vi "ReadJSONImageAcquisitionParameters.vi"(8 "error in":errorcluster, 10 "Camera ID":string="0", 11 "file path (use dialog)":path) -> (0 "error out":errorcluster, 3 "Camera parameters":T1 {"Camera parameters"."Image Type" items=["Grayscale (U8)", "Grayscale (I16)", "Grayscale (SGL)", "Complex (CSG)", "RGB (U32)", "HSL (U32)", "RGB (U64)", "Grayscale (U16)"]})   [LabVIEW 2019, in "Image Acquisition.lvlib" / "Image Acquisition.lvclass"]
uses:
  Image Acquisition.lvclass
  <vilib>/userdefined/High Color/IMAQdx.ctl
  <vilib>/vision/driver/IMAQdx.llb/IMAQdx Acquisition Mode.ctl
  <vilib>/vision/driver/IMAQdx.llb/IMAQdx Buffer Number Mode.ctl
  TypeDefs/Image Acquisition Parameters JSON.ctl
  TypeDefs/Image Acquisition Parameters.ctl
panel:
  out "VCluster\n out":variant
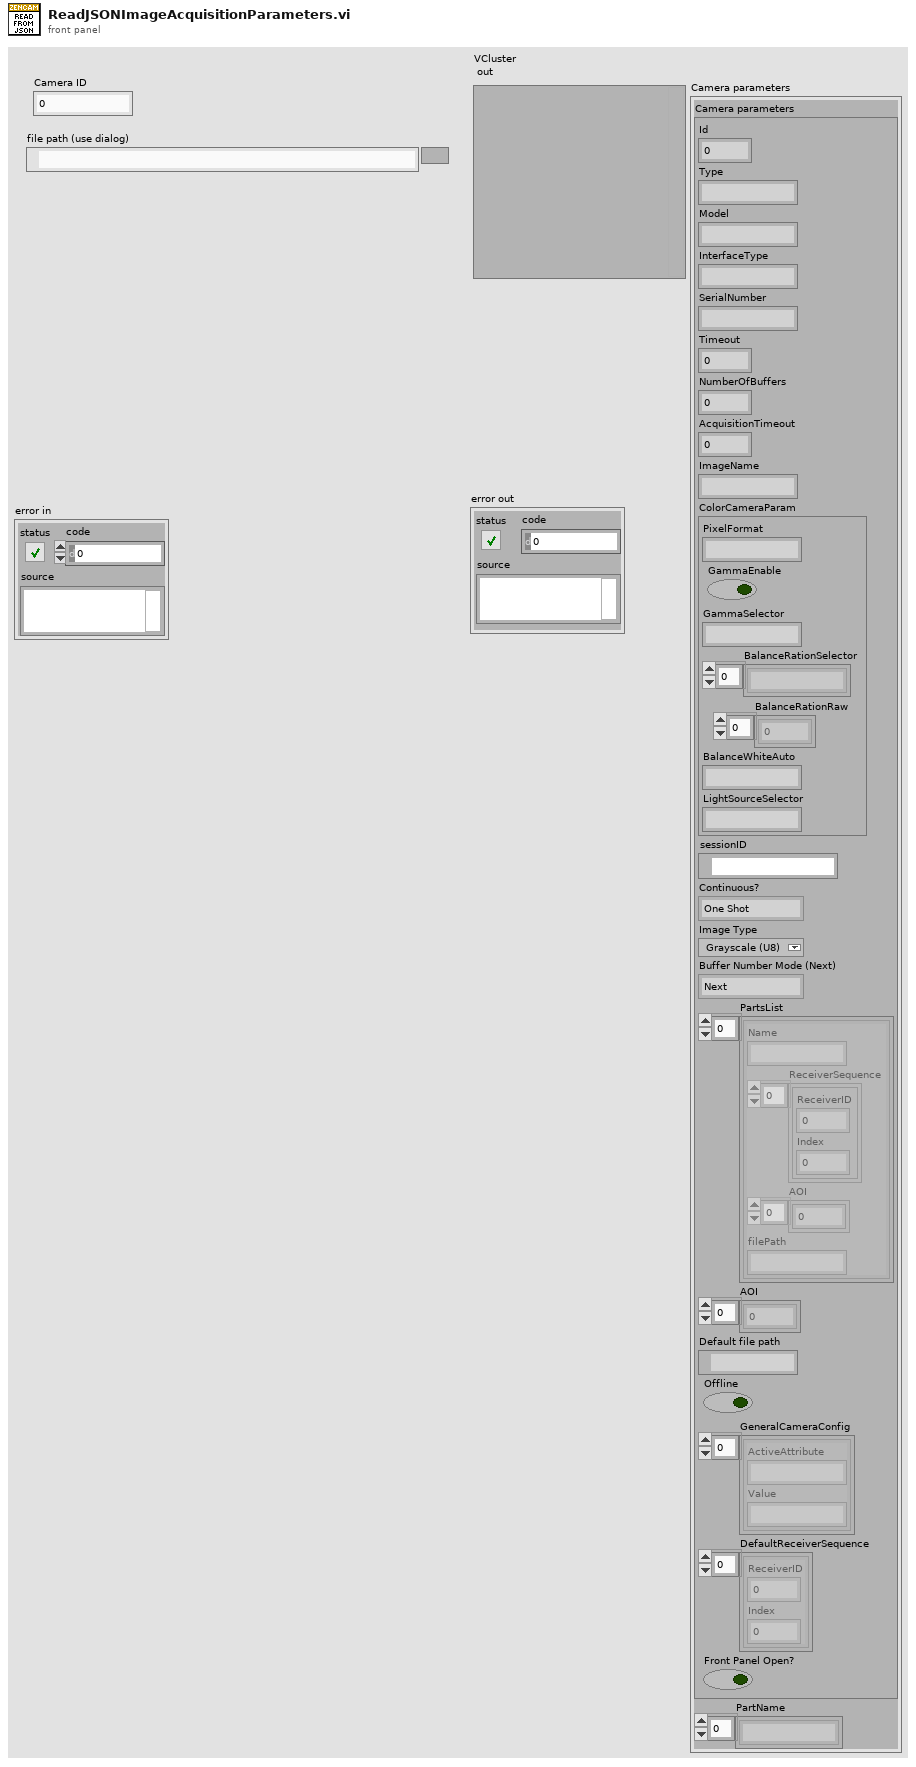
[diagram p1: front panel]
types:
  T1 = typedef "Image Acquisition.lvlib/Image Acquisition.lvclass/Image Acquisition Parameters.ctl" = cluster{"Camera parameters":cluster{"Id":i32, "Type":string, "Model":string, "InterfaceType":string, "SerialNumber":string, "Timeout":i32, "NumberOfBuffers":i32, "AcquisitionTimeout":i32, "ImageName":string, "ColorCameraParam":cluster{"PixelFormat":string, "GammaEnable":bool, "GammaSelector":string, "BalanceRationSelector":string[], "BalanceRationRaw":i32[], "BalanceWhiteAuto":string, "LightSourceSelector":string}, "sessionID":T2, "Continuous?":T3, "Image Type":T4, "Buffer Number Mode (Next)":T5, "PartsList":cluster{"Name":string, "ReceiverSequence":cluster{"ReceiverID":dbl, "Index":dbl}[], "AOI":i32[], "filePath":string}[], "AOI ":i32[], "Default file path":path, "Offline":bool, "GeneralCameraConfig":cluster{"ActiveAttribute":string, "Value":string}[], "DefaultReceiverSequence":cluster{"ReceiverID":dbl, "Index":dbl}[], "Front Panel Open?":bool}, "PartName":string[]}
  T2 = typedef "IMAQdx.ctl" = refnum<k21>
  T3 = typedef "NI_Vision_Acquisition_Software.lvlib/IMAQdx Acquisition Mode.ctl" = enum32{"One Shot", "Continuous"}
  T4 = typedef "Image Type" = u32
  T5 = typedef "NI_Vision_Acquisition_Software.lvlib/IMAQdx Buffer Number Mode.ctl" = enum32{"Next", "Last", "Buffer Number", "Every", "Last New"}
  T6 = typedef "Image Acquisition.lvlib/Image Acquisition.lvclass/Image Acquisition Parameters JSON.ctl" = cluster{"Image Acquisition Paramters":cluster{"Id":i32, "SessionID":string, "Type":string, "Model":string, "InterfaceType":string, "SerialNumber":string, "Timeout":i32, "GeneralCameraConfig":cluster{"ActiveAttribute":string, "Value":string}[], "DefaultAOI":i32[], "DefaultReceiverSequence":cluster{"ReceiverID":i32, "Index":i32}[], "DefaultfileName":string, "Continuous":i32, "NumberOfBuffers":i32, "BufferNumberMode":i32, "acquisitionTimeout":i32, "ImageType":i32, "Offline":bool, "FrontPanelOpen":bool, "ColorCameraParam":cluster{"PixelFormat":string, "GammaEnable":bool, "GammaSelector":string, "BalanceRationSelector":string[], "BalanceRationRaw":i32[], "BalanceWhiteAuto":string, "LightSourceSelector":string}, "PartsList":cluster{"Name":string, "ReceiverSequence":cluster{"ReceiverID":i32, "Index":i32}[], "AOI":i32[], "filePath":string}[]}, "PartName":string[]}
  T7 = cluster{"ActiveAttribute":string, "Value":string}[]
  T8 = cluster{"PixelFormat":string, "GammaEnable":bool, "GammaSelector":string, "BalanceRationSelector":string[], "BalanceRationRaw":i32[], "BalanceWhiteAuto":string, "LightSourceSelector":string}
  T9 = cluster{"Name":string, "ReceiverSequence":cluster{"ReceiverID":i32, "Index":i32}[], "AOI":i32[], "filePath":string}[]
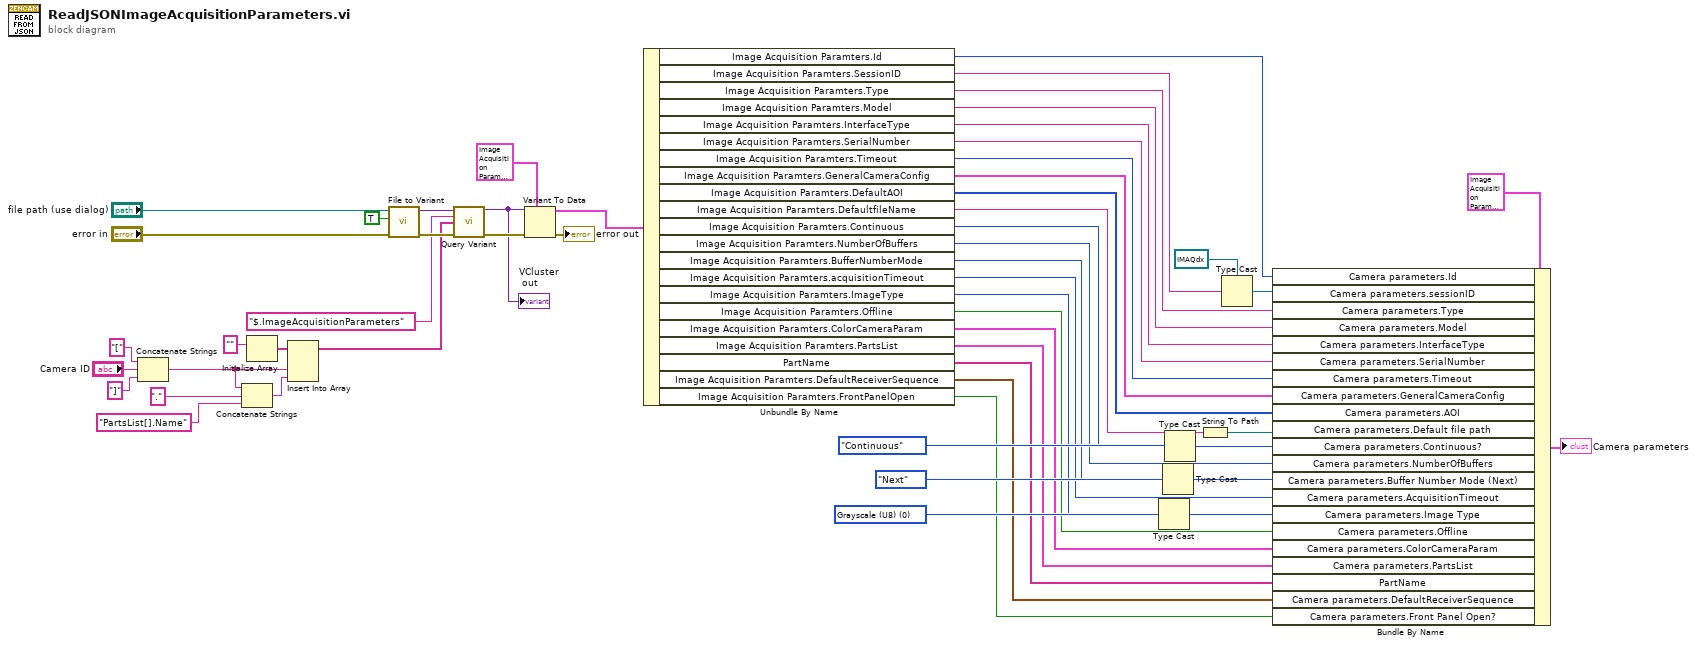
[diagram p0: block diagram]
diagram:
  w46 = T4 0 items=["Grayscale (U8)", "Grayscale (I16)", "Grayscale (SGL)", "Complex (CSG)", "RGB (U32)", "HSL (U32)", "RGB (U64)", "Grayscale (U16)"] ("Image Type")
  n1 = Concatenate Strings("[" ("string"), "Camera ID", "]" ("string")) -> (w39:string)
  n2 = Concatenate Strings(w39, "." ("string"), "PartsList[].Name" ("new element/subarray")) -> (w36:string)
  n3 = Initialize Array("") -> (w43:string[])  [unwired: 1 in]
  n4 = Insert Into Array(array=w43, new element #1=w39, new element #2=w36) -> (w1:string[])  [unwired: 1 in]
  n5 = call <vilib>:"File to Variant.vi"("JSON FilePath"="file path (use dialog)", "Remove Comments?"=TRUE, "error in (no error)"="error in") -> ("JSON Variant"=w3:variant, "error out"=w6:errorcluster)  [unwired: 5 in, 1 out]
  n6 = call <vilib>:"Query Variant.vi"("VCluster in"=w3, "basePath in"="$.ImageAcquisitionParameters", "pathList"=w1, "error IO"=w6) -> ("VCluster\n out"=w4:variant, "error out"=w5:errorcluster)  [unwired: 8 in, 2 out]
  "VCluster\n out" <- w4
  n7 = Variant To Data(error in=w5, type=T6 {"Image Acquisition Paramters"={"Id"=0, "SessionID"="", "Type"="", "Model"="", "InterfaceType"="", "SerialNumber"="", "Timeout"=0, "GeneralCameraConfig"=[], "DefaultAOI"=[], "DefaultReceiverSequence"=[], "DefaultfileName"="", "Continuous"=0, "NumberOfBuffers"=0, "BufferNumberMode"=0, "acquisitionTimeout"=0, "ImageType"=0, "Offline"=FALSE, "FrontPanelOpen"=FALSE, "ColorCameraParam"={"PixelFormat"="", "GammaEnable"=FALSE, "GammaSelector"="", "BalanceRationSelector"=[], "BalanceRationRaw"=[], "BalanceWhiteAuto"="", "LightSourceSelector"=""}, "PartsList"=[]}, "PartName"=[]} ("Cluster"), Variant=w4) -> (data=w30:T6, error out=→"error out":errorcluster)
  n8 = Unbundle By Name(w30) -> ("Image Acquisition Paramters.Id"=w29:i32, "Image Acquisition Paramters.SessionID"=w52:string, "Image Acquisition Paramters.Type"=w51:string, "Image Acquisition Paramters.Model"=w50:string, "Image Acquisition Paramters.InterfaceType"=w49:string, "Image Acquisition Paramters.SerialNumber"=w48:string, "Image Acquisition Paramters.Timeout"=w28:i32, "Image Acquisition Paramters.GeneralCameraConfig"=w27:T7, "Image Acquisition Paramters.DefaultAOI"=w26:i32[], "Image Acquisition Paramters.DefaultfileName"=w24:string, "Image Acquisition Paramters.Continuous"=w23:i32, "Image Acquisition Paramters.NumberOfBuffers"=w21:i32, "Image Acquisition Paramters.BufferNumberMode"=w20:i32, "Image Acquisition Paramters.acquisitionTimeout"=w18:i32, "Image Acquisition Paramters.ImageType"=w16:i32, "Image Acquisition Paramters.Offline"=w15:bool, "Image Acquisition Paramters.ColorCameraParam"=w14:T8, "Image Acquisition Paramters.PartsList"=w13:T9, "PartName"=w12:string[], "Image Acquisition Paramters.DefaultReceiverSequence"=w11:cluster{"ReceiverID":i32, "Index":i32}[], "Image Acquisition Paramters.FrontPanelOpen"=w10:bool)
  n9 = Type Cast(type=w46, x=w16) -> (*(type *) &x=w17:T4)
  n10 = Type Cast(type=IMAQdx_Buffer_Number_Mode."Next" ("Buffer Number Mode (Next)"), x=w20) -> (*(type *) &x=w19:T5)
  n11 = Type Cast(type=IMAQdx_Acquisition_Mode."Continuous" ("Continuous?"), x=w23) -> (*(type *) &x=w22:T3)
  n12 = String To Path(string=w24) -> (path=w25:path)
  n13 = Type Cast(type=T2 refnum ("Imaqdx Session In"), x=w52) -> (*(type *) &x=w32:T2)
  n14 = Bundle By Name(cluster=T1 {"Camera parameters"={"Id"=0, "Type"="", "Model"="", "InterfaceType"="", "SerialNumber"="", "Timeout"=0, "NumberOfBuffers"=0, "AcquisitionTimeout"=0, "ImageName"="", "ColorCameraParam"={"PixelFormat"="", "GammaEnable"=FALSE, "GammaSelector"="", "BalanceRationSelector"=[], "BalanceRationRaw"=[], "BalanceWhiteAuto"="", "LightSourceSelector"=""}, "sessionID"="", "Continuous?"=enum."One Shot", "Image Type"=0, "Buffer Number Mode (Next)"=enum."Next", "PartsList"=[], "AOI "=[], "Default file path"=path "", "Offline"=FALSE, "GeneralCameraConfig"=[], "DefaultReceiverSequence"=[], "Front Panel Open?"=FALSE}, "PartName"=[]} ("Camera parameters"), "Camera parameters.Id"=w29, "Camera parameters.sessionID"=w32, "Camera parameters.Type"=w51, "Camera parameters.Model"=w50, "Camera parameters.InterfaceType"=w49, "Camera parameters.SerialNumber"=w48, "Camera parameters.Timeout"=w28, "Camera parameters.GeneralCameraConfig"=w27, "Camera parameters.AOI"=w26, "Camera parameters.Default file path"=w25, "Camera parameters.Continuous?"=w22, "Camera parameters.NumberOfBuffers"=w21, "Camera parameters.Buffer Number Mode (Next)"=w19, "Camera parameters.AcquisitionTimeout"=w18, "Camera parameters.Image Type"=w17, "Camera parameters.Offline"=w15, "Camera parameters.ColorCameraParam"=w14, "Camera parameters.PartsList"=w13, "PartName"=w12, "Camera parameters.DefaultReceiverSequence"=w11, "Camera parameters.Front Panel Open?"=w10) -> (→"Camera parameters":T1)
